vi "movingpoint.vi"(4 "Fine Down":bool, 6 "Fine Up":bool, 7 "Buttons":bool[](array[boolean]), 8 "Pot Scaled Value":dbl, 9 "Setpoints":dbl[](array[numeric]), 10 "Setpoint Index":i32, 11 "MotorControlDevRef":T1={"DeviceStatus"={"status"=FALSE, "code"=0, "source"=""}, "Type"=enum."PWM", "PWM"={"Controller"=enum."Controller 1", "PWM Channel"=enum."Invalid", "DeadBand"={"Name"="", "maxPositivePwm"=0, "minPositivePwm"=0, "centerPwm"=0, "maxNegativePwm"=0, "minNegativePwm"=0, "angularRange"=0}}, "CAN"={"Device Number"=0, "Control Mode"=enum."Percent VBus", "Semaphore"=refnum, "Max Vout"=12.0, "TalonSRX Control Mode"=enum."Percent VBus"}, "Invert"=FALSE, "TransformRef"=refnum, "InvTransformRef"=refnum}) -> (3 "Stopped":bool=TRUE)   [LabVIEW 2014]
uses:
  <vilib>/Rock Robotics/WPI/MotorControl/WPI_MotorControlDeviceRef.ctl
  <vilib>/Rock Robotics/WPI/MotorControl/WPI_MotorControlType.ctl
  <vilib>/Rock Robotics/SystemInterfaces/Typedef/FPGA_TypedefDigitalModule.ctl
  <vilib>/Rock Robotics/SystemInterfaces/DIO/FPGA_DIOPWMChannel.ctl
  <vilib>/Rock Robotics/WPI/PWM/WPI_PWMDeadband.ctl
  <vilib>/Rock Robotics/WPI/CAN/Jaguar/SubVIs/WPI_CANJaguar_ControlMode.ctl
  <vilib>/Rock Robotics/WPI/CAN/TalonSRX/WPI_CANTalonSRX_APIControlMode.ctl
  <vilib>/Rock Robotics/WPI/PWM/WPI_PWMTransform_ConPane.ctl
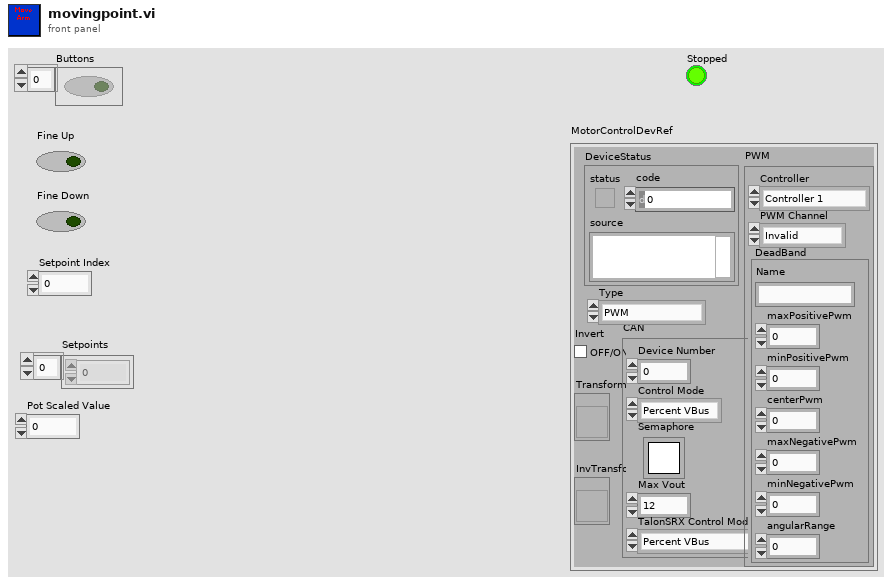
[diagram p1: front panel]
types:
  T1 = typedef "WPI_MotorControlDeviceRef.ctl" = cluster{"DeviceStatus":errorcluster, "Type":T2, "PWM":cluster{"Controller":T3, "PWM Channel":T4, "DeadBand":T5}, "CAN":cluster{"Device Number":u8, "Control Mode":T6, "Semaphore":T7, "Max Vout":dbl, "TalonSRX Control Mode":T8}, "Invert":bool, "TransformRef":T9, "InvTransformRef":T9}
  T2 = typedef "WPI_MotorControlType.ctl" = enum16{"PWM", "CAN", "CANTalonSRX"}
  T3 = typedef "FPGA_TypedefDigitalModule.ctl" = enum16{"Controller 1"}
  T4 = typedef "FPGA_DIOPWMChannel.ctl" = enum8{"PWM 0", "PWM 1", "PWM 2", "PWM 3", "PWM 4", "PWM 5", "PWM 6", "PWM 7", "PWM 8", "PWM 9", "PWM MXP 0", "PWM MXP 1", "PWM MXP 2", "PWM MXP 3", "PWM MXP 4", "PWM MXP 5", "PWM MXP 6", "PWM MXP 7", "PWM MXP 8", "PWM MXP 9", "Invalid"}
  T5 = typedef "WPI_PWMDeadband.ctl" = cluster{"Name":string, "maxPositivePwm":i32, "minPositivePwm":i32, "centerPwm":i32, "maxNegativePwm":i32, "minNegativePwm":i32, "angularRange":u16}
  T6 = typedef "WPI_CANJaguar_ControlMode.ctl" = enum8{"Percent VBus", "Current", "Speed", "Position", "Voltage"}
  T7 = typedef "Semaphore RefNum" = refnum<k1>
  T8 = typedef "WPI_CANTalonSRX_APIControlMode.ctl" = enum8{"Percent VBus", "Speed", "Position", "Slave", "Unchanged / Invalid"}
  T9 = typedef "WPI_PWMTransform_ConPane.ctl" = refnum<vi>
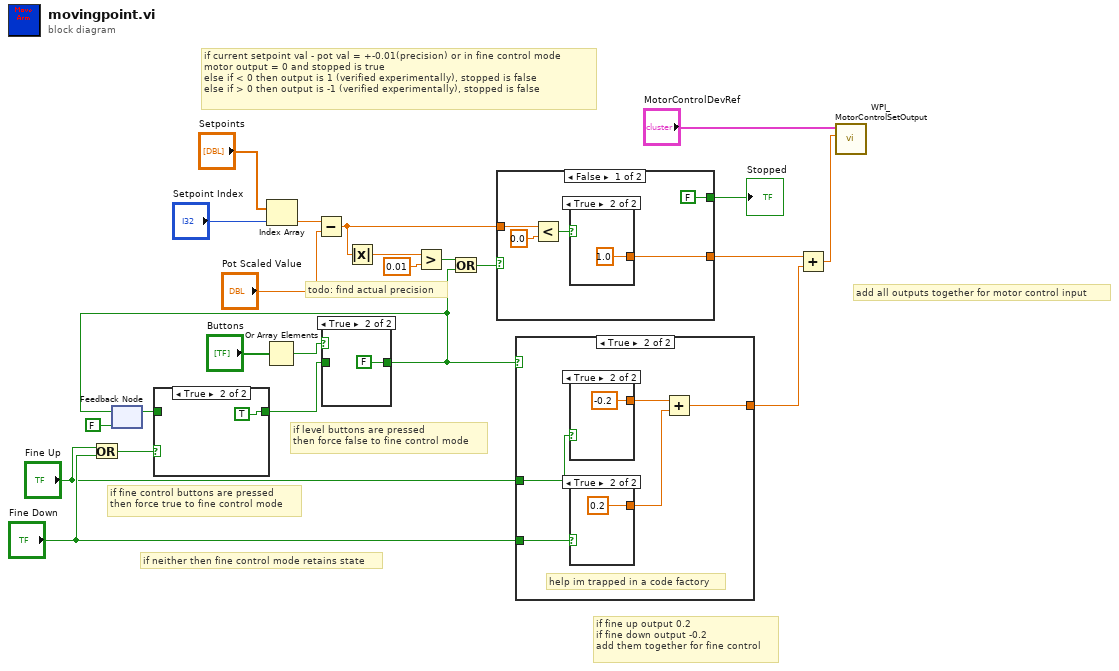
[diagram p0: block diagram]
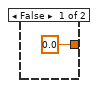
[diagram p2: hidden frame]
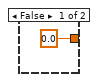
[diagram p3: hidden frame]
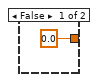
[diagram p4: hidden frame]
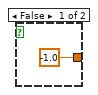
[diagram p7: hidden frame]
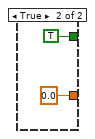
[diagram p8: hidden frame]
diagram:
  # "add all outputs together for motor control input"
  # "if fine up output 0.2\nif fine down output -0.2\nadd them together for fine control"
  # "if neither then fine control mode retains state"
  # "if fine control buttons are pressed\nthen force true to fine control mode"
  # "if level buttons are pressed\nthen force false to fine control mode"
  # "todo: find actual precision"
  # "if current setpoint val - pot val = +-0.01(precision) or in fine control mode \nmotor output = 0 and stopped is true\nelse if < 0 then output is 1 (verified experimentally), stopped is false\nelse if > 0 then output is -1 (verified experimentally), stopped is false"
  n1 = Or(x="Fine Up", y="Fine Down") -> (x .or. y?=w11:bool)
  n2 = feedback #1(FALSE) -> (w10:bool)
  n3 = case shown="True" w11 {
    tunnel: w10 -> [w24 _]
    tunnel: [w24 TRUE] -> w9
    frame False {
    }
    frame True {
    }
  }
  n4 = Or Array Elements(Boolean array="Buttons") -> (logical OR=w13:bool)
  n5 = Index Array(array="Setpoints", index="Setpoint Index") -> (element=w21:dbl)
  n6 = Subtract(x=w21, y="Pot Scaled Value") -> (x-y=w17:dbl)
  n7 = case shown="True" w13 {
    tunnel: [w26 FALSE] -> w2
    tunnel: w9 -> [w26 _]
    frame False {
    }
    frame True {
    }
  }
  n8 = feedback-in #1(w2) -> ()
  n9 = Absolute Value(x=w17) -> (abs(x)=w18:dbl)
  n10 = Greater?(x=w18, y=0.01) -> (0:w3:bool)
  n11 = Or(x=w3, y=w2) -> (x .or. y?=w1:bool)
  n12 = case shown="False" w1 {
    tunnel: [w32 0.0] -> w6
    tunnel: w17 -> [w29 _]
    tunnel: [FALSE TRUE] -> w16
    frame False {
      n13 = Less?(x=w29, y=0.0) -> (x < y?=w31:bool)
      n14 = case shown="True" w31 {
        tunnel: [-1.0 1.0] -> w32
        frame False {
        }
        frame True {
        }
      }
    }
    frame True {
    }
  }
  "Stopped" <- w16
  n15 = case shown="True" w2 {
    tunnel: "Fine Down" -> [_ w42]
    tunnel: "Fine Up" -> [_ w41]
    tunnel: [0.0 w38] -> w5
    frame False {
    }
    frame True {
      # "help im trapped in a code factory"
      n16 = case shown="True" w41 {
        tunnel: [0.0 -0.2] -> w40
        frame False {
        }
        frame True {
        }
      }
      n17 = case shown="True" w42 {
        tunnel: [0.0 0.2] -> w39
        frame False {
        }
        frame True {
        }
      }
      n18 = Add(x=w40, y=w39) -> (x+y=w38:dbl)
    }
  }
  n19 = Add(x=w6, y=w5) -> (x+y=w4:dbl)
  n20 = call <vilib>:"WPI_MotorControlSetOutput.vi"("Output"=w4, "MotorControlDevRef"="MotorControlDevRef") -> ()  [unwired: 7 in, 3 out]
